vi "openRefsMain.vi"(8 "error in (no error)":errorcluster {"code" format="Error %.0f"}, 11 "objectRefsMain":T1) -> (0 "error out":errorcluster {"code" format="Error %.0f"}, 2 "GObjectsFound":i32, 3 "objectRefsMainOut":T1, 4 "FPobjectLabels":string[][](array[string]))   [LabVIEW 2017]
doc: "This VI opens the calling (or parent) VIs FP control, pane, and spitter refnums programatically and builds them into a cluster of GObject Refnums."
uses:
  Controls/objectRefsMain.ctl
  <vilib>/Utility/error.llb/Error Cluster From Error Code.vi
  <vilib>/ErrorRing/Error Ring.xnode
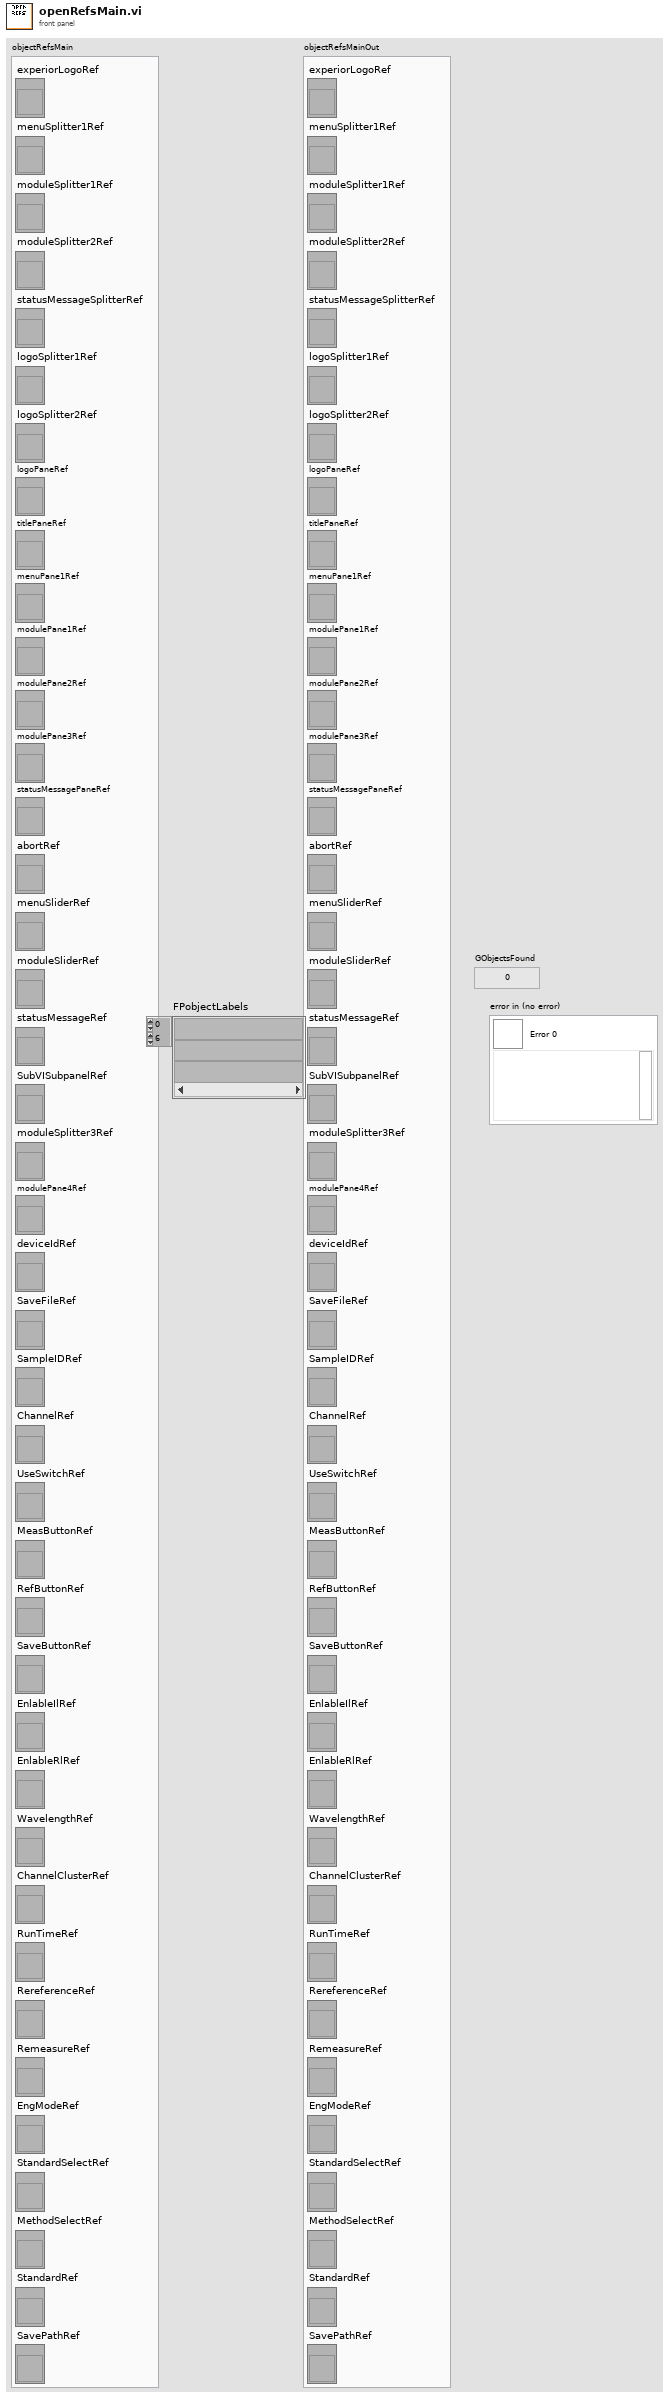
[diagram p1: front panel]
types:
  T1 = typedef "objectRefsMain.ctl" = cluster{"experiorLogoRef":refnum<vi>, "menuSplitter1Ref":refnum<vi>, "moduleSplitter1Ref":refnum<vi>, "moduleSplitter2Ref":refnum<vi>, "statusMessageSplitterRef":refnum<vi>, "logoSplitter1Ref":refnum<vi>, "logoSplitter2Ref":refnum<vi>, "logoPaneRef":refnum<vi>, "titlePaneRef":refnum<vi>, "menuPane1Ref":refnum<vi>, "modulePane1Ref":refnum<vi>, "modulePane2Ref":refnum<vi>, "modulePane3Ref":refnum<vi>, "statusMessagePaneRef":refnum<vi>, "abortRef":refnum<vi>, "menuSliderRef":refnum<vi>, "moduleSliderRef":refnum<vi>, "statusMessageRef":refnum<vi>, "SubVISubpanelRef":refnum<vi>, "moduleSplitter3Ref":refnum<vi>, "modulePane4Ref":refnum<vi>, "deviceIdRef":refnum<vi>, "SaveFileRef":refnum<vi>, "SampleIDRef":refnum<vi>, "ChannelRef":refnum<vi>, "UseSwitchRef":refnum<vi>, "MeasButtonRef":refnum<vi>, "RefButtonRef":refnum<vi>, "SaveButtonRef":refnum<vi>, "EnlableIlRef":refnum<vi>, "EnlableRlRef":refnum<vi>, "WavelengthRef":refnum<vi>, "ChannelClusterRef":refnum<vi>, "RunTimeRef":refnum<vi>, "RereferenceRef":refnum<vi>, "RemeasureRef":refnum<vi>, "EngModeRef":refnum<vi>, "StandardSelectRef":refnum<vi>, "MethodSelectRef":refnum<vi>, "StandardRef":refnum<vi>, "SavePathRef":refnum<vi>}
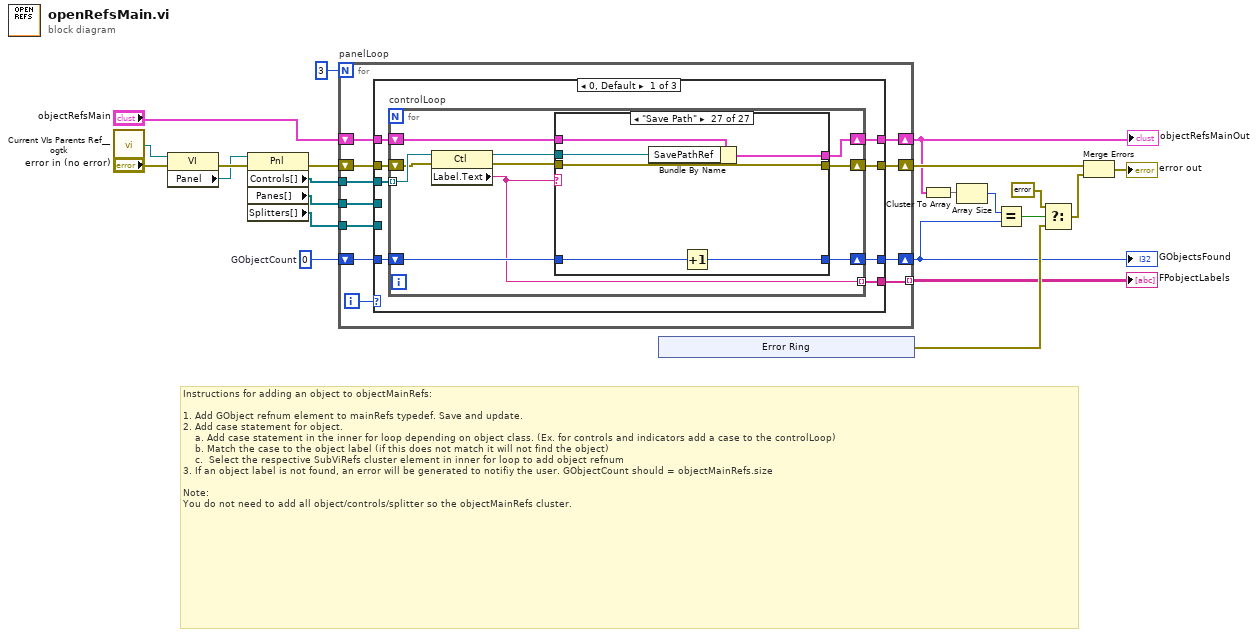
[diagram p0: block diagram]
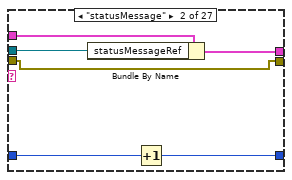
[diagram p3: hidden frame]
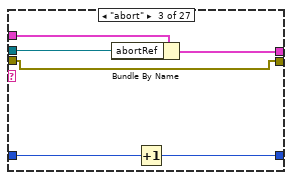
[diagram p4: hidden frame]
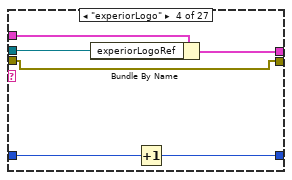
[diagram p5: hidden frame]
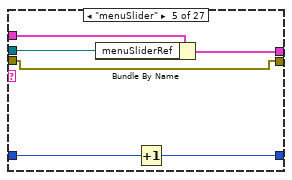
[diagram p6: hidden frame]
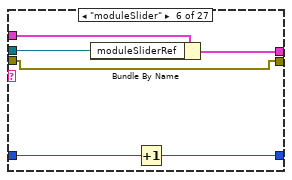
[diagram p7: hidden frame]
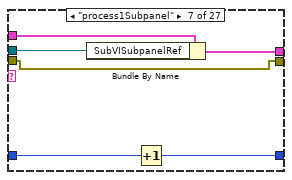
[diagram p8: hidden frame]
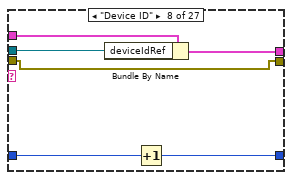
[diagram p9: hidden frame]
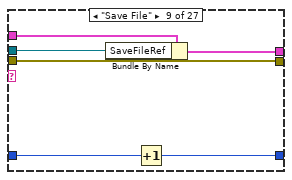
[diagram p10: hidden frame]
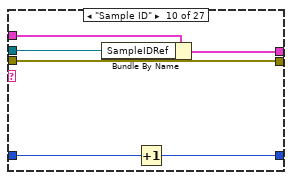
[diagram p11: hidden frame]
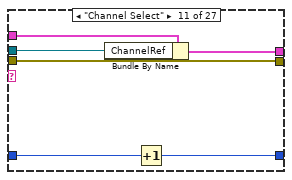
[diagram p12: hidden frame]
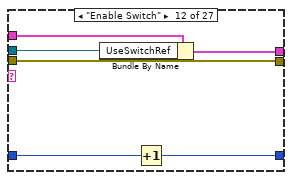
[diagram p13: hidden frame]
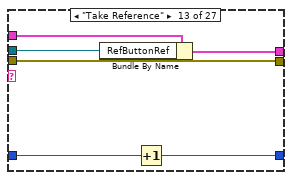
[diagram p14: hidden frame]
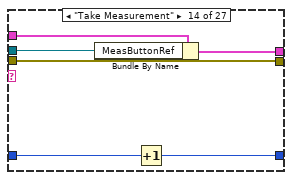
[diagram p15: hidden frame]
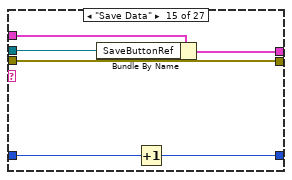
[diagram p16: hidden frame]
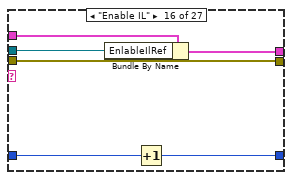
[diagram p17: hidden frame]
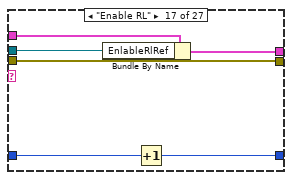
[diagram p18: hidden frame]
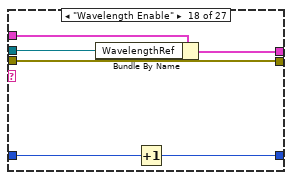
[diagram p19: hidden frame]
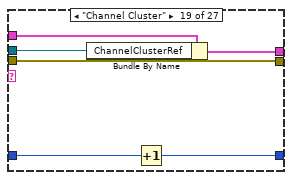
[diagram p20: hidden frame]
diagram:
  w14 = 0  # GObjectCount
  # "Instructions for adding an object to objectMainRefs:\n\n1. Add GObject refnum element to mainRefs typedef. Save and update.\n2. Add case statement for object.\n    a. Add case statement in the inner for loop depending on object class. (Ex. for controls and indicators add a case to the controlLoop)\n    b. Match the case to the object label (if this does not match it will not find the object)\n    c.  Select the respective SubViRefs cluster element in inner for loop to add object refnum\n3. If an object label is not found, an error will be generated to notifiy the user. GObjectCount should = objectMainRefs.size\n\nNote: \nYou do not need to add all object/controls/splitter so the objectMainRefs cluster."
  n1 = call <userlib>:"Current VIs Parents Ref__ogtk.vi"() -> ("Calling VI's Reference"=w6:refnum<vi>)  [unwired: 2 in]
  n2 = property class="VI"(reference=w6, error in="error in (no error)") -> (error out=w21:errorcluster, "Panel"=w19:refnum<vi>)  [unwired: 1 out]
  n3 = property class="Pnl"(reference=w19, error in=w21) -> (error out=w20:errorcluster, "Controls[]"=w15:refnum<vi>[], "Panes[]"=w17:refnum<vi>[], "Splitters[]"=w16:refnum<vi>[])  [unwired: 1 out]
  n4 = for "panelLoop" {
    N: 3 -> [_]
    tunnel: w15 -> [w33]
    shift-right: [w31] -> w8
    shift-left: w20 -> [w32]
    shift-right: [w29] -> w3
    shift-left: "objectRefsMain" -> [w30]
    tunnel: w17 -> [w27]
    tunnel: w16 -> [w26]
    shift-right: [w24] -> w1
    shift-left: w14 -> [w25]
    tunnel: [w23] -> w4 mode=indexing
    i -> [w28]
    n5 = case shown="0, Default" w28 {
      tunnel: w33 -> [w41 w219 w289]
      tunnel: w32 -> [w40 w218 w288]
      tunnel: [w39 w217 w287] -> w31
      tunnel: w30 -> [w38 w216 w286]
      tunnel: [w37 w215 w285] -> w29
      tunnel: w27 -> [_ w214 _]
      tunnel: w26 -> [_ _ w284]
      tunnel: w25 -> [w36 w213 w283]
      tunnel: [w35 w212 w282] -> w24
      tunnel: [w34 w211 w281] -> w23
      frame 0, Default {
        n6 = for "controlLoop" {
          tunnel: w41 -> [w51] mode=indexing
          shift-right: [w46] -> w39
          shift-left: w40 -> [w49]
          shift-right: [w45] -> w37
          shift-left: w38 -> [w48]
          shift-right: [w43] -> w35
          shift-left: w36 -> [w44]
          tunnel: [w42] -> w34 mode=indexing
          n7 = property class="Ctl"(reference=w51, error in=w49) -> (reference out=w50:refnum<vi>, error out=w47:errorcluster, "Label.Text"=w42:string)
          n8 = case shown="\"Save Path\"" w42 {
            tunnel: w50 -> [_ w58 w64 w70 w76 w82 w88 w94 w100 w106 w112 w118 w124 w130 w136 w142 w148 w154 w160 w166 w172 w178 w184 w190 w196 w202 w208]
            tunnel: w48 -> [w54 w60 w66 w72 w78 w84 w90 w96 w102 w108 w114 w120 w126 w132 w138 w144 w150 w156 w162 w168 w174 w180 w186 w192 w198 w204 w210]
            tunnel: [w54 w59 w65 w71 w77 w83 w89 w95 w101 w107 w113 w119 w125 w131 w137 w143 w149 w155 w161 w167 w173 w179 w185 w191 w197 w203 w209] -> w45
            tunnel: w47 -> [w53 w57 w63 w69 w75 w81 w87 w93 w99 w105 w111 w117 w123 w129 w135 w141 w147 w153 w159 w165 w171 w177 w183 w189 w195 w201 w207]
            tunnel: [w53 w57 w63 w69 w75 w81 w87 w93 w99 w105 w111 w117 w123 w129 w135 w141 w147 w153 w159 w165 w171 w177 w183 w189 w195 w201 w207] -> w46
            tunnel: w44 -> [w52 w56 w62 w68 w74 w80 w86 w92 w98 w104 w110 w116 w122 w128 w134 w140 w146 w152 w158 w164 w170 w176 w182 w188 w194 w200 w206]
            tunnel: [w52 w55 w61 w67 w73 w79 w85 w91 w97 w103 w109 w115 w121 w127 w133 w139 w145 w151 w157 w163 w169 w175 w181 w187 w193 w199 w205] -> w43
            frame Default {
              # "IL/RL Array Initialized in data:fromSubVI"
            }
            frame "statusMessage" {
              n9 = Bundle By Name(cluster=w60, "statusMessageRef"=w58) -> (w59:T1)
              n10 = Increment(x=w56) -> (x+1=w55:i32)
            }
            frame "abort" {
              n11 = Bundle By Name(cluster=w66, "abortRef"=w64) -> (w65:T1)
              n12 = Increment(x=w62) -> (x+1=w61:i32)
            }
            frame "experiorLogo" {
              n13 = Bundle By Name(cluster=w72, "experiorLogoRef"=w70) -> (w71:T1)
              n14 = Increment(x=w68) -> (x+1=w67:i32)
            }
            frame "menuSlider" {
              n15 = Bundle By Name(cluster=w78, "menuSliderRef"=w76) -> (w77:T1)
              n16 = Increment(x=w74) -> (x+1=w73:i32)
            }
            frame "moduleSlider" {
              n17 = Bundle By Name(cluster=w84, "moduleSliderRef"=w82) -> (w83:T1)
              n18 = Increment(x=w80) -> (x+1=w79:i32)
            }
            frame "process1Subpanel" {
              n19 = Bundle By Name(cluster=w90, "SubVISubpanelRef"=w88) -> (w89:T1)
              n20 = Increment(x=w86) -> (x+1=w85:i32)
            }
            frame "Device ID" {
              n21 = Bundle By Name(cluster=w96, "deviceIdRef"=w94) -> (w95:T1)
              n22 = Increment(x=w92) -> (x+1=w91:i32)
            }
            frame "Save File" {
              n23 = Bundle By Name(cluster=w102, "SaveFileRef"=w100) -> (w101:T1)
              n24 = Increment(x=w98) -> (x+1=w97:i32)
            }
            frame "Sample ID" {
              n25 = Bundle By Name(cluster=w108, "SampleIDRef"=w106) -> (w107:T1)
              n26 = Increment(x=w104) -> (x+1=w103:i32)
            }
            frame "Channel Select" {
              n27 = Bundle By Name(cluster=w114, "ChannelRef"=w112) -> (w113:T1)
              n28 = Increment(x=w110) -> (x+1=w109:i32)
            }
            frame "Enable Switch" {
              n29 = Bundle By Name(cluster=w120, "UseSwitchRef"=w118) -> (w119:T1)
              n30 = Increment(x=w116) -> (x+1=w115:i32)
            }
            frame "Take Reference" {
              n31 = Bundle By Name(cluster=w126, "RefButtonRef"=w124) -> (w125:T1)
              n32 = Increment(x=w122) -> (x+1=w121:i32)
            }
            frame "Take Measurement" {
              n33 = Bundle By Name(cluster=w132, "MeasButtonRef"=w130) -> (w131:T1)
              n34 = Increment(x=w128) -> (x+1=w127:i32)
            }
            frame "Save Data" {
              n35 = Bundle By Name(cluster=w138, "SaveButtonRef"=w136) -> (w137:T1)
              n36 = Increment(x=w134) -> (x+1=w133:i32)
            }
            frame "Enable IL" {
              n37 = Bundle By Name(cluster=w144, "EnlableIlRef"=w142) -> (w143:T1)
              n38 = Increment(x=w140) -> (x+1=w139:i32)
            }
            frame "Enable RL" {
              n39 = Bundle By Name(cluster=w150, "EnlableRlRef"=w148) -> (w149:T1)
              n40 = Increment(x=w146) -> (x+1=w145:i32)
            }
            frame "Wavelength Enable" {
              n41 = Bundle By Name(cluster=w156, "WavelengthRef"=w154) -> (w155:T1)
              n42 = Increment(x=w152) -> (x+1=w151:i32)
            }
            frame "Channel Cluster" {
              n43 = Bundle By Name(cluster=w162, "ChannelClusterRef"=w160) -> (w161:T1)
              n44 = Increment(x=w158) -> (x+1=w157:i32)
            }
            frame "Running" {
              n45 = Bundle By Name(cluster=w168, "RunTimeRef"=w166) -> (w167:T1)
              n46 = Increment(x=w164) -> (x+1=w163:i32)
            }
            frame "Rereference" {
              n47 = Bundle By Name(cluster=w174, "RereferenceRef"=w172) -> (w173:T1)
              n48 = Increment(x=w170) -> (x+1=w169:i32)
            }
            frame "Remeasure" {
              n49 = Bundle By Name(cluster=w180, "RemeasureRef"=w178) -> (w179:T1)
              n50 = Increment(x=w176) -> (x+1=w175:i32)
            }
            frame "Engineering Mode" {
              n51 = Bundle By Name(cluster=w186, "EngModeRef"=w184) -> (w185:T1)
              n52 = Increment(x=w182) -> (x+1=w181:i32)
            }
            frame "Standard Selection" {
              n53 = Bundle By Name(cluster=w192, "StandardSelectRef"=w190) -> (w191:T1)
              n54 = Increment(x=w188) -> (x+1=w187:i32)
            }
            frame "Method Selection" {
              n55 = Bundle By Name(cluster=w198, "MethodSelectRef"=w196) -> (w197:T1)
              n56 = Increment(x=w194) -> (x+1=w193:i32)
            }
            frame "IL RL Standards" {
              n57 = Bundle By Name(cluster=w204, "StandardRef"=w202) -> (w203:T1)
              n58 = Increment(x=w200) -> (x+1=w199:i32)
            }
            frame "Save Path" {
              n59 = Bundle By Name(cluster=w210, "SavePathRef"=w208) -> (w209:T1)
              n60 = Increment(x=w206) -> (x+1=w205:i32)
            }
          }
        }
      }
      frame 1 {
        n61 = for "paneLoop" {
          tunnel: w219 -> [_] mode=indexing
          shift-right: [w225] -> w217
          shift-left: w218 -> [w228]
          shift-right: [w224] -> w215
          shift-left: w216 -> [w227]
          shift-right: [w222] -> w212
          shift-left: w213 -> [w223]
          tunnel: w214 -> [w221] mode=indexing
          tunnel: [w220] -> w211 mode=indexing
          n62 = property class="Pane"(reference=w221, error in=w228) -> (reference out=w229:refnum<vi>, error out=w226:errorcluster, "Label.Text"=w220:string)
          n63 = case shown="\"modulePane1\"" w220 {
            tunnel: w229 -> [_ w236 w242 w248 w254 w260 w266 w272 w278]
            tunnel: w227 -> [w232 w238 w244 w250 w256 w262 w268 w274 w280]
            tunnel: [w232 w237 w243 w249 w255 w261 w267 w273 w279] -> w224
            tunnel: w226 -> [w231 w235 w241 w247 w253 w259 w265 w271 w277]
            tunnel: [w231 w235 w241 w247 w253 w259 w265 w271 w277] -> w225
            tunnel: w223 -> [w230 w234 w240 w246 w252 w258 w264 w270 w276]
            tunnel: [w230 w233 w239 w245 w251 w257 w263 w269 w275] -> w222
            frame Default {
            }
            frame "logoPane" {
              n64 = Bundle By Name(cluster=w238, "logoPaneRef"=w236) -> (w237:T1)
              n65 = Increment(x=w234) -> (x+1=w233:i32)
            }
            frame "titlePane" {
              n66 = Bundle By Name(cluster=w244, "titlePaneRef"=w242) -> (w243:T1)
              n67 = Increment(x=w240) -> (x+1=w239:i32)
            }
            frame "menuPane1" {
              n68 = Bundle By Name(cluster=w250, "menuPane1Ref"=w248) -> (w249:T1)
              n69 = Increment(x=w246) -> (x+1=w245:i32)
            }
            frame "modulePane1" {
              n70 = Bundle By Name(cluster=w256, "modulePane1Ref"=w254) -> (w255:T1)
              n71 = Increment(x=w252) -> (x+1=w251:i32)
            }
            frame "modulePane2" {
              n72 = Bundle By Name(cluster=w262, "modulePane2Ref"=w260) -> (w261:T1)
              n73 = Increment(x=w258) -> (x+1=w257:i32)
            }
            frame "modulePane3" {
              n74 = Bundle By Name(cluster=w268, "modulePane3Ref"=w266) -> (w267:T1)
              n75 = Increment(x=w264) -> (x+1=w263:i32)
            }
            frame "modulePane4" {
              n76 = Bundle By Name(cluster=w274, "modulePane4Ref"=w272) -> (w273:T1)
              n77 = Increment(x=w270) -> (x+1=w269:i32)
            }
            frame "statusMessagePane" {
              n78 = Bundle By Name(cluster=w280, "statusMessagePaneRef"=w278) -> (w279:T1)
              n79 = Increment(x=w276) -> (x+1=w275:i32)
            }
          }
        }
      }
      frame 2 {
        n80 = for "splitterLoop" {
          tunnel: w289 -> [_] mode=indexing
          shift-right: [w295] -> w287
          shift-left: w288 -> [w298]
          shift-right: [w294] -> w285
          shift-left: w286 -> [w297]
          shift-right: [w292] -> w282
          shift-left: w283 -> [w293]
          tunnel: w284 -> [w291] mode=indexing
          tunnel: [w290] -> w281 mode=indexing
          n81 = property class="Splitter"(reference=w291, error in=w298) -> (reference out=w299:refnum<vi>, error out=w296:errorcluster, "Label.Text"=w290:string)
          n82 = case shown="\"moduleSplitter1\"" w290 {
            tunnel: w299 -> [_ w306 w312 w318 w324 w330 w336 w342]
            tunnel: w297 -> [w302 w308 w314 w320 w326 w332 w338 w344]
            tunnel: [w302 w307 w313 w319 w325 w331 w337 w343] -> w294
            tunnel: w296 -> [w301 w305 w311 w317 w323 w329 w335 w341]
            tunnel: [w301 w305 w311 w317 w323 w329 w335 w341] -> w295
            tunnel: w293 -> [w300 w304 w310 w316 w322 w328 w334 w340]
            tunnel: [w300 w303 w309 w315 w321 w327 w333 w339] -> w292
            frame Default {
            }
            frame "statusMessageSplitter" {
              n83 = Bundle By Name(cluster=w308, "statusMessageSplitterRef"=w306) -> (w307:T1)
              n84 = Increment(x=w304) -> (x+1=w303:i32)
            }
            frame "logoSplitter1" {
              n85 = Bundle By Name(cluster=w314, "logoSplitter1Ref"=w312) -> (w313:T1)
              n86 = Increment(x=w310) -> (x+1=w309:i32)
            }
            frame "logoSplitter2" {
              n87 = Bundle By Name(cluster=w320, "logoSplitter2Ref"=w318) -> (w319:T1)
              n88 = Increment(x=w316) -> (x+1=w315:i32)
            }
            frame "menuSplitter1" {
              n89 = Bundle By Name(cluster=w326, "menuSplitter1Ref"=w324) -> (w325:T1)
              n90 = Increment(x=w322) -> (x+1=w321:i32)
            }
            frame "moduleSplitter1" {
              n91 = Bundle By Name(cluster=w332, "moduleSplitter1Ref"=w330) -> (w331:T1)
              n92 = Increment(x=w328) -> (x+1=w327:i32)
            }
            frame "moduleSplitter2" {
              n93 = Bundle By Name(cluster=w338, "moduleSplitter2Ref"=w336) -> (w337:T1)
              n94 = Increment(x=w334) -> (x+1=w333:i32)
            }
            frame "moduleSplitter3" {
              n95 = Bundle By Name(cluster=w344, "moduleSplitter3Ref"=w342) -> (w343:T1)
              n96 = Increment(x=w340) -> (x+1=w339:i32)
            }
          }
        }
      }
    }
  }
  "GObjectsFound" <- w1
  "objectRefsMainOut" <- w3
  "FPobjectLabels" <- w4
  n97 = xnode "Error Ring"() -> ("error out"=w9:errorcluster)
  n98 = Cluster To Array(cluster=w3) -> (array=w2:refnum<vi>[])
  n99 = Array Size(array=w2) -> (size(s)=w13:i32)
  n100 = Equal?(x=w13, y=w1) -> (x = y?=w12:bool)
  n101 = Select(t=errorcluster {"status"=FALSE, "code"=0, "source"=""} ("error in (no error)"), s=w12, f=w9) -> (s? t:f=w10:errorcluster)
  n102 = Merge Errors(w8, w10) -> (→"error out":errorcluster)
